vi "HFRR ADV v07.vi"() -> ()   [LabVIEW 2025] (continued)
    n1256 = property on="FF Calibration g" class="WFGraph (strict)"("Visible"=w1675) -> ()  [unwired: 2 in, 2 out]
    n1257 = property on="Lift" class="Bool (strict)"("Visible"=w1675) -> ()  [unwired: 2 in, 2 out]
    n1258 = property on="Threshold" class="DigNum (strict)"("Visible"=w1675) -> ()  [unwired: 2 in, 2 out]
    n1259 = property on="Time slide" class="Slide (strict)"("Visible"=w1675) -> ()  [unwired: 2 in, 2 out]
    n1260 = call "Elapsed Time2"("Time Target (s)"=w1686, "Auto Reset"=TRUE) -> ("Time has Elapsed"=w1676:bool)  [unwired: 10 in, 7 out]
    n1261 = case shown="True" w1676 {
      frame False {
        # "79.77669138"
        # "2.3554"
        n1262 = local read "FRIC. FORCE :"() -> (w1739:dbl)
        n1263 = local read "FF cal val"() -> (w1736:dbl[])
        n1264 = Multiply(x=w1739, y=79.77669138) -> (x*y=w1738:dbl)
        n1265 = Multiply(x=w1736, y=w1738) -> (x*y=→"FF Calibration g":dbl[])
        "Err Count" <- 0 ("y")
      }
      frame True {
        n1266 = stacked-sequence {
          frame #0 {
            n1267 = stacked-sequence {
              frame #0 {
                "Lift" <- TRUE ("Lift")
              }
            }
          }
          frame #1 {
            w1751 = 2500 ("y")
            n1268 = local read "RUN"() -> (w1743:bool)
            n1269 = local read "FF1"() -> (w1746:dbl[])
            n1270 = case shown="False" w1743 {
              frame False {
                n1271 = local write "Frequency"(0.0 ("Frequency")) -> ()
              }
              frame True {
              }
            }
            n1272 = Array Size(array=w1746) -> (size(s)=w1745:i32)
            n1273 = local read "Ch1"() -> (w1742:dbl[])
            "Waveform Chart 2" <- w1742
            n1274 = call-poly <vilib>:"Mean.vi"("X"=w1742) -> ("mean"=→"Raw Mean":dbl)  [unwired: 1 out]
            n1275 = Insert Into Array(array=w1746, index=w1745, new element=w1742) -> (w1748:dbl[])
            n1276 = Array Size(array=w1748) -> (size(s)=w1752:i32)
            n1277 = Subtract(x=w1752, y=w1751) -> (x-y=w1750:i32)
            n1278 = Greater?(x=w1752, y=w1751) -> (0:w1753:bool)
            n1279 = case shown="True" w1753 {
              tunnel: w1750 -> [_ w1757]
              tunnel: [w1755 w1759] -> w1744
              tunnel: w1748 -> [w1755 w1758]
              frame False {
              }
              frame True {
                n1280 = Delete From Array(array=w1758, length=w1757, index=0) -> (array with subset deleted=w1759:dbl[])  [unwired: 1 out]
                "Numeric" <- w1757
              }
            }
            "FF1" <- w1744
            "PID Ref" <- TRUE ("PID Ref")
          }
          frame #2 {
          }
          frame #3 {
            w1767 = 0.0 ("lower limit")
            # "CONVERT TO N"
            # "DATA PROCESSING"
            # "115 mV/N"
            n1281 = local read "RH Numeric:"() -> (w1761:dbl)
            n1282 = local read "HUMIDITY:"() -> (w1762:dbl)
            n1283 = local read "temp buf"() -> (w1825:dbl[])
            n1284 = local read "Air temp"() -> (w1823:dbl[])
            n1285 = local read "ecr buf"() -> (w1784:dbl[])
            n1286 = local read "Fric Val"() -> (w1829:dbl[])
            n1287 = case shown="True" "Boolean 5" {
              frame False {
              }
              frame True {
                n1288 = local write "Boolean 5"(FALSE) -> ()
                n1289 = local write "Captured Values"(dbl[][] [] ("Captured Values")) -> ()
                n1290 = local write "Best Fit"(dbl[] [] ("Best Fit")) -> ()
              }
            }
            n1291 = local read "TEMPERATURE :"() -> (w1806:dbl)
            n1292 = call-poly <vilib>:"Mean.vi"("X"=w1784) -> ("mean"=w1781:dbl)  [unwired: 1 out]
            n1293 = call-poly <vilib>:"Mean.vi"("X"=w1823) -> ("mean"=w1791:dbl)  [unwired: 1 out]
            "Raw air temp" <- w1791
            n1294 = call-poly <vilib>:"Mean.vi"("X"=w1825) -> ("mean"=w1793:dbl)  [unwired: 1 out]
            "Raw specimen temp" <- w1793
            n1295 = local read "TEMP INTERCEPT:"() -> (w1798:dbl)
            n1296 = Multiply(x=w1761, y=w1762) -> (x*y=→"Humidity ( %RH )" →"Hum" →"Hum 2":dbl)
            n1297 = Multiply(x=w1829, y=1.0) -> (x*y=w1830:dbl[])
            n1298 = local read "FRIC. FORCE :"() -> (w1822:dbl)
            n1299 = Multiply(x=w1793, y=w1806) -> (x*y=w1787:dbl)
            n1300 = local read "AIR TEMPERATURE :"() -> (w1807:dbl)
            n1301 = local read "RUN"() -> (w1819:bool)
            n1302 = Add(x=w1791, y="Offset Air Temp") -> (x+y=w1786:dbl)
            n1303 = local read "AIR TEMP INTERCEPT:"() -> (w1803:dbl)
            n1304 = case shown="0, Default" "Calibrating" {
              tunnel: w1793 -> [w1849 _]
              tunnel: [w1849 w1850] -> w1792
              tunnel: w1791 -> [_ w1850]
              frame 0, Default {
              }
              frame 1 {
              }
            }
            n1305 = Multiply(x=w1781, y="ECR_Gain") -> (x*y=w1780:dbl)
            n1306 = Add(x=w1787, y=w1798) -> (x+y=w1804:dbl)
            n1307 = Multiply(x=w1822, y=79.77669138) -> (x*y=w1820:dbl)
            n1308 = Select(t=0.01 ("FF fil1"), s=w1819, f=0.1 ("FF fil1")) -> (s? t:f=w1815:dbl)
            n1309 = local read "ecr"() -> (w1775:dbl)
            n1310 = Multiply(x=w1786, y=w1807) -> (x*y=w1788:dbl)
            n1311 = Multiply(x=w1830, y=w1820) -> (x*y=w1827:dbl[])
            n1312 = Multiply(x=w1780, y=0.2) -> (x*y=w1773:dbl)
            n1313 = Multiply(x=0.8, y=w1775) -> (x*y=w1774:dbl)
            n1314 = call <vilib>:"Mean PtByPt.vi"("x"=w1804, "sample length"=10) -> ("mean"=w1763:dbl)  [unwired: 2 in, 1 out]
            "TEMP 2" <- w1763
            "TEMP 3" <- w1763
            n1315 = local read "AIR TEMP"() -> (w1812:dbl)
            n1316 = Add(x=w1788, y=w1803) -> (x+y=w1805:dbl)
            n1317 = call-poly <vilib>:"Mean.vi"("X"=w1827) -> ("mean"=w1828:dbl)  [unwired: 1 out]
            n1318 = Add(x=w1773, y=w1774) -> (x+y=w1772:dbl)
            n1319 = Subtract(x=1.0 ("y"), y=w1815) -> (x-y=w1813:dbl)
            n1320 = local write "TEMP"(w1763) -> ()
            n1321 = Multiply(x=w1813, y=w1812) -> (x*y=w1811:dbl)
            n1322 = Multiply(x=w1805, y=w1815) -> (x*y=w1816:dbl)
            n1323 = Not A Number/Path/Refnum?(number/path/refnum=w1772) -> (NaN/Path/Refnum?=w1782:bool)
            n1324 = Subtract(x=w1827, y=w1828) -> (x-y=w1797:dbl[])
            n1325 = local read "FRICVALZ"() -> (w1837:dbl)
            n1326 = case shown="True" "Boolean 4" {
              tunnel: w1792 -> [_ w1856]
              tunnel: "Standard Temp. ( °c )" -> [_ w1855]
              frame False {
              }
              frame True {
                n1327 = Build Array(w1855, w1856) -> (w1854:dbl[])
                n1328 = local write "Boolean 4"(FALSE ("Boolean 4")) -> ()
                n1329 = local read "Captured Values"() -> (w1853:dbl[][])
                n1330 = Build Array (concatenate)(w1853, w1854) -> (w1851:dbl[][])
                n1331 = local write "Captured Values"(w1851) -> ()
              }
            }
            n1332 = Or(x="FRICVALZ 3", y="FRICVALZ 2") -> (x .or. y?=w1765:bool)
            n1333 = Add(x=w1816, y=w1811) -> (x+y=w1809:dbl)
            n1334 = Absolute Value(x=w1797) -> (abs(x)=w1832:dbl[])
            n1335 = call-poly <vilib>:"RMS.vi"("X"=w1797) -> ("rms value"=w1796:dbl)  [unwired: 1 out]
            n1336 = Select(t=0.0, s=w1782, f=w1772) -> (s? t:f=w1779:dbl)
            n1337 = call-poly <vilib>:"Mean.vi"("X"=w1832) -> ()  [unwired: 2 out]
            n1338 = local read "FF 2"() -> (w1839:dbl)
            n1339 = case shown="True" w1765 {
              tunnel: w1796 -> [_ w1861]
              frame False {
              }
              frame True {
                w1860 = FALSE ("FRICVALZ")
                n1340 = local write "FRICVALZ 3"(w1860) -> ()
                n1341 = local write "FRICVALZ 2"(w1860) -> ()
                "FRICVALZ" <- w1861
              }
            }
            n1342 = Subtract(x=w1796, y=w1837) -> (x-y=w1831:dbl)
            n1343 = Not A Number/Path/Refnum?(number/path/refnum=w1809) -> (NaN/Path/Refnum?=w1810:bool)
            n1344 = In Range and Coerce(upper limit=100.0, x=w1779, lower limit=w1767) -> ()  [unwired: 2 out]
            n1345 = Select(t=0.0, s=w1810, f=w1809) -> (s? t:f=w1769:dbl)
            "AIR TEMP" <- w1769
            n1346 = Multiply(x=w1831, y=0.1 ("FF fil1")) -> (x*y=w1843:dbl)
            n1347 = Multiply(x=0.9 ("FF fil2"), y=w1839) -> (x*y=w1842:dbl)
            n1348 = call "Elapsed Time11"("Time Target (s)"=1.0) -> ("Time has Elapsed"=w1771:bool)  [unwired: 11 in, 7 out]
            n1349 = Add(x=w1843, y=w1842) -> (x+y=w1766:dbl)
            "FF 2" <- w1766
            "FF 4" <- w1766
            n1350 = local read "NORMAL LOAD"() -> (w1826:dbl)
            n1351 = case shown="True" w1771 {
              tunnel: w1769 -> [_ w1845]
              frame False {
              }
              frame True {
                "AirT" <- w1845
              }
            }
            n1352 = local read "TEMP"() -> (w1836:dbl)
            n1353 = Not A Number/Path/Refnum?(number/path/refnum=w1766) -> (NaN/Path/Refnum?=w1834:bool)
            n1354 = Divide(x=w1766, y=w1826) -> (x/y=w1799:dbl)
            n1355 = Not A Number/Path/Refnum?(number/path/refnum=w1836) -> (NaN/Path/Refnum?=w1835:bool)
            n1356 = Compound Arithmetic op=OR(w1835, w1834) -> (w1833:bool)
            n1357 = Not A Number/Path/Refnum?(number/path/refnum=w1799) -> (NaN/Path/Refnum?=w1801:bool)
            n1358 = case shown="True" w1833 {
              frame False {
              }
              frame True {
                n1359 = local write "TEMP"(0.0 ("TEMP")) -> ()
                n1360 = local write "FF 2"(0.0 ("FF 2")) -> ()
                n1361 = local write "reinit"(TRUE ("reinit")) -> ()
              }
            }
            n1362 = Select(t=0.0, s=w1801, f=w1799) -> (s? t:f=→"COF 2":dbl)
            "ecr" <- w1767
          }
          frame #4 {
            n1363 = flat-sequence {
              frame #0 {
                n1364 = Wait (ms)(milliseconds to wait=u32 100) -> ()  [unwired: 1 out]
              }
              frame #1 {
                n1365 = local write "Lift"(FALSE ("Lift")) -> ()
              }
            }
            n1366 = case shown="True" "Boolean 6" {
              frame False {
              }
              frame True {
                n1367 = local write "Boolean 6"(FALSE ("Boolean 6")) -> ()
                n1368 = local read "Captured Values"() -> (w1872:dbl[][])
                n1369 = Index Array(array=w1872, index (col) #1=0 ("disabled index (col)"), index (col) #2=1 ("index (col)")) -> (element #1=w1870:dbl[], element #2=w1868:dbl[])  [unwired: 2 in]
                n1370 = call <vilib>:"Linear Fit.vi"("Y"=w1870, "X"=w1868) -> ("Best Linear Fit"=→"Best Fit":dbl[], "slope"=w1864:dbl, "intercept"=w1863:dbl)  [unwired: 9 in, 2 out]
                "Slope" <- w1864
                "Intercept" <- w1863
                n1371 = local read "Calibrating"() -> (w1865:u16)
                n1372 = case shown="1" w1865 {
                  tunnel: w1864 -> [w1874 w1876]
                  tunnel: w1863 -> [w1873 w1875]
                  frame 0, Default {
                    n1373 = local write "TEMPERATURE :"(w1874) -> ()
                    n1374 = local write "TEMP INTERCEPT:"(w1873) -> ()
                  }
                  frame 1 {
                    n1375 = local write "AIR TEMPERATURE :"(w1876) -> ()
                    n1376 = local write "AIR TEMP INTERCEPT:"(w1875) -> ()
                  }
                }
              }
            }
          }
        }
      }
    }
    n1377 = Wait (ms)(milliseconds to wait=u32 50) -> ()  [unwired: 1 out]
    n1378 = local read "Quit"() -> (w1667:bool)
    "Rate" <- 2500.0 ("No of Samples")
    "Humid Last buf" <- dbl[] [0.0, 0.0, 0.0, 0.0] ("Humid Last buf")
  }
  n1379 = while {
    tunnel: w53 -> [_]
    tunnel: [w1906] -> _
    tunnel: [w1881] -> w50
    i -> [w1906]
    stop <- w1881 stop-if-true
    # "C:\\LAB-IQ-NXT\\Scar View.exe"
    n1380 = local read "OK Button 16"() -> (w1895:bool)
    n1381 = local read "Re-Initialise"() -> (w1891:bool)
    n1382 = local read "Main Tab"() -> (w1887:T3)
    n1383 = local read "service 3"() -> (w1888:bool)
    n1384 = local read "OPEN 6"() -> (w1890:bool)
    n1385 = local read "EDIT 2"() -> (w1893:bool)
    n1386 = flat-sequence {
      frame #0 {
        n1387 = stacked-sequence {
          frame #0 {
            n1388 = local read "EDIT"() -> (w2560:bool)
            n1389 = case shown="True" w2560 {
              tunnel: [u8 2 ("Disabled") u8 0 ("Disabled")] -> _
              frame False {
                w2562 = FALSE
                n1390 = local write "Password"("") -> ()
                n1391 = property on="SrvM CP" class="Bool (strict)"("Visible"=w2562) -> ()  [unwired: 2 in, 2 out]
                n1392 = property on="message" class="Str"("Visible"=w2562) -> ()  [unwired: 2 in, 2 out]
                n1393 = local write "x = y?"(w2562) -> ()
                n1394 = property on="Password" class="Str"("Visible"=w2562) -> ()  [unwired: 2 in, 2 out]
                n1395 = property on="ENTER THE NEW PASSWORD" class="Str"("Visible"=w2562) -> ()  [unwired: 2 in, 2 out]
                n1396 = property on="ENTER CURRENT PASSWORD" class="Str"("Visible"=w2562) -> ()  [unwired: 2 in, 2 out]
                n1397 = local write "SrvM CP"(w2562) -> ()
              }
              frame True {
                w2565 = TRUE
                n1398 = property on="SrvM CP" class="Bool (strict)"("Visible"=w2565) -> ()  [unwired: 2 in, 2 out]
                n1399 = property on="Password" class="Str"("Visible"=w2565) -> ()  [unwired: 2 in, 2 out]
              }
            }
            "dipl pwd" <- "@143$\n" ("dipl pwd")
          }
          frame #1 {
            # "Gain password"
            n1400 = String To Byte Array(string="ENTER CURRENT PASSWORD") -> (unsigned byte array=w2570:u8[])
            n1401 = Search 1D Array(1D array=w2570, element=u8 10) -> (index of element=w2573:i32)  [unwired: 1 in]
            n1402 = Index Array(array=w2570, index=w2573) -> (element=w2569:u8)
            n1403 = Equal?(x=w2569, y=10) -> (x = y?=w2567:bool)
            n1404 = case shown="True" w2567 {
              frame False {
                n1405 = property on="ENTER THE NEW PASSWORD" class="Str"("Visible"=FALSE) -> ()  [unwired: 2 in, 2 out]
              }
              frame True {
                # "password"
                # "change password logic"
                n1406 = local read "ENTER CURRENT PASSWORD"() -> (w2586:string)
                n1407 = local read "dipl pwd"() -> (w2580:string)
                n1408 = String To Byte Array(string=w2586) -> (unsigned byte array=w2588:u8[])
                n1409 = String To Byte Array(string=w2580) -> (unsigned byte array=w2581:u8[])
                n1410 = Array Size(array=w2588) -> (size(s)=w2585:i32)
                n1411 = Array Size(array=w2581) -> (size(s)=w2583:i32)
                n1412 = for {
                  N: w2585 -> [_]
                  tunnel: w2588 -> [w2612]
                  tunnel: [w2610] -> w2589 mode=indexing
                  tunnel: w2585 -> [w2604]
                  i -> [w2605]
                  n1413 = Decrement(x=w2604) -> (x-1=w2602:i32)
                  n1414 = Equal?(x=w2605, y=w2602) -> (x = y?=w2603:bool)
                  n1415 = Index Array(array=w2612, index=w2605) -> (element=w2606:u8)
                  n1416 = Number To Decimal String(number=w2606) -> (decimal integer string=w2611:string)  [unwired: 1 in]
                  n1417 = Select(t="", s=w2603, f="\r") -> (s? t:f=w2608:string)
                  n1418 = Concatenate Strings(w2611, w2608) -> (w2610:string)
                }
                n1419 = for {
                  N: w2583 -> [_]
                  tunnel: w2581 -> [w2600]
                  tunnel: [w2598] -> w2582 mode=indexing
                  tunnel: w2583 -> [w2595]
                  i -> [w2596]
                  n1420 = Decrement(x=w2595) -> (x-1=w2594:i32)
                  n1421 = Equal?(x=w2596, y=w2594) -> (x = y?=w2593:bool)
                  n1422 = Index Array(array=w2600, index=w2596) -> (element=w2599:u8)
                  n1423 = Number To Decimal String(number=w2599) -> (decimal integer string=w2597:string)  [unwired: 1 in]
                  n1424 = Select(t="", s=w2593, f="\r") -> (s? t:f=w2590:string)
                  n1425 = Concatenate Strings(w2597, w2590) -> (w2598:string)
                }
                n1426 = local read "string"() -> (w2587:string)
                n1427 = Concatenate Strings(w2582) -> (w2576:string)
                n1428 = Concatenate Strings(w2587) -> (w2584:string)
                n1429 = Concatenate Strings(w2589) -> (w2577:string)
                n1430 = Equal?(x=w2577, y=w2584) -> (x = y?=w2579:bool)
                n1431 = Equal?(x=w2577, y=w2576) -> (x = y?=w2575:bool)
                n1432 = Or(x=w2579, y=w2575) -> (x .or. y?=w2578:bool)
                n1433 = case shown="True" w2578 {
                  frame False {
                  }
                  frame True {
                    n1434 = property on="ENTER THE NEW PASSWORD" class="Str"("Visible"=TRUE) -> ()  [unwired: 2 in, 2 out]
                  }
                }
              }
            }
          }
          frame #2 {
            n1435 = String To Byte Array(string="ENTER THE NEW PASSWORD") -> (unsigned byte array=w2615:u8[])
            n1436 = Search 1D Array(1D array=w2615, element=u8 10) -> (index of element=w2619:i32)  [unwired: 1 in]
            n1437 = Index Array(array=w2615, index=w2619) -> (element=w2617:u8)
            n1438 = Equal?(x=w2617, y=10) -> (x = y?=w2614:bool)
            n1439 = case shown="False" w2614 {
              frame False {
              }
              frame True {
                n1440 = local write "EDIT"(FALSE) -> ()
                n1441 = local write "SrvM CP"(FALSE) -> ()
                n1442 = local read "ENTER THE NEW PASSWORD"() -> (w2622:string)
                n1443 = String To Byte Array(string=w2622) -> (unsigned byte array=w2627:u8[])
                n1444 = Array Size(array=w2627) -> (size(s)=w2624:i32)
                n1445 = for {
                  N: w2624 -> [_]
                  tunnel: w2627 -> [w2640]
                  tunnel: [w2637] -> w2629 mode=indexing
                  tunnel: w2624 -> [w2632]
                  i -> [w2630]
                  n1446 = Decrement(x=w2632) -> (x-1=w2633:i32)
                  n1447 = Equal?(x=w2630, y=w2633) -> (x = y?=w2634:bool)
                  n1448 = Index Array(array=w2640, index=w2630) -> (element=w2639:u8)
                  n1449 = Number To Decimal String(number=w2639) -> (decimal integer string=w2638:string)  [unwired: 1 in]
                  n1450 = Select(t="", s=w2634, f="\r") -> (s? t:f=w2631:string)
                  n1451 = Concatenate Strings(w2638, w2631) -> (w2637:string)
                }
                n1452 = local read "file path"() -> (w2621:path)
                n1453 = Concatenate Strings(w2629) -> (w2623:string)
                n1454 = Delete(path (use dialog)=w2621) -> (deleted path=w2625:path)  [unwired: 4 in, 2 out]
                n1455 = call <vilib>:"Write Characters To File.vi"("append to file? (new file:F)"=FALSE, "character string"=w2623, "file path (dialog if empty)"=w2625) -> ()  [unwired: 2 in, 1 out]
              }
            }
          }
          frame #3 {
            n1456 = case shown="True" "SrvM CP" {
              frame False {
                w2643 = ""
                n1457 = local write "ENTER CURRENT PASSWORD"(w2643) -> ()
                n1458 = local write "ENTER THE NEW PASSWORD"(w2643) -> ()
                n1459 = property on="ENTER CURRENT PASSWORD" class="Str"("Visible"=FALSE) -> ()  [unwired: 2 in, 2 out]
              }
              frame True {
                n1460 = property on="ENTER THE NEW PASSWORD" class="Str"() -> ("Visible"=w2644:bool)  [unwired: 2 in, 2 out]
                n1461 = Not(x=w2644) -> (.not. x?=w2645:bool)
                n1462 = property on="ENTER CURRENT PASSWORD" class="Str"("Visible"=w2645) -> ()  [unwired: 2 in, 2 out]
              }
            }
          }
          frame #4 {
            n1463 = String To Byte Array(string="Password") -> (unsigned byte array=w2652:u8[])
            n1464 = Search 1D Array(1D array=w2652, element=u8 10) -> (index of element=w2650:i32)  [unwired: 1 in]
            n1465 = Index Array(array=w2652, index=w2650) -> (element=w2651:u8)
            n1466 = Equal?(x=w2651, y=10) -> (x = y?=w2647:bool)
            n1467 = case shown="True" w2647 {
              frame False {
              }
              frame True {
                # "password"
                # "password"
                n1468 = local read "Password"() -> (w2665:string)
                n1469 = String To Byte Array(string=w2665) -> (unsigned byte array=w2668:u8[])
                n1470 = String To Byte Array(string="@143$\n") -> (unsigned byte array=w2654:u8[])
                n1471 = Array Size(array=w2668) -> (size(s)=w2663:i32)
                n1472 = Array Size(array=w2654) -> (size(s)=w2659:i32)
                n1473 = for {
                  N: w2663 -> [_]
                  tunnel: w2668 -> [w2685]
                  tunnel: [w2683] -> w2669 mode=indexing
                  tunnel: w2663 -> [w2680]
                  i -> [w2681]
                  n1474 = Decrement(x=w2680) -> (x-1=w2679:i32)
                  n1475 = Index Array(array=w2685, index=w2681) -> (element=w2684:u8)
                  n1476 = Equal?(x=w2681, y=w2679) -> (x = y?=w2678:bool)
                  n1477 = Number To Decimal String(number=w2684) -> (decimal integer string=w2682:string)  [unwired: 1 in]
                  n1478 = Select(t="", s=w2678, f="\r") -> (s? t:f=w2675:string)
                  n1479 = Concatenate Strings(w2682, w2675) -> (w2683:string)
                }
                n1480 = for {
                  N: w2659 -> [_]
                  tunnel: w2654 -> [w2696]
                  tunnel: [w2694] -> w2657 mode=indexing
                  tunnel: w2659 -> [w2691]
                  i -> [w2692]
                  n1481 = Decrement(x=w2691) -> (x-1=w2690:i32)
                  n1482 = Index Array(array=w2696, index=w2692) -> (element=w2695:u8)
                  n1483 = Equal?(x=w2692, y=w2690) -> (x = y?=w2689:bool)
                  n1484 = Number To Decimal String(number=w2695) -> (decimal integer string=w2693:string)  [unwired: 1 in]
                  n1485 = Select(t="", s=w2689, f="\r") -> (s? t:f=w2686:string)
                  n1486 = Concatenate Strings(w2693, w2686) -> (w2694:string)
                }
                n1487 = local read "file path"() -> (w2653:path)
                n1488 = call <vilib>:"Read Characters From File.vi"("file path (dialog if empty)"=w2653) -> ("character string"=w2667:string)  [unwired: 5 in, 3 out]
                "string" <- w2667
                n1489 = flat-sequence {
                  tunnel: [w2670] -> w2664
                  frame #0 {
                    w2670 = ""
                    n1490 = local write "Password"(w2670) -> ()
                  }
                }
                n1491 = Concatenate Strings(w2657) -> (w2658:string)
                n1492 = Concatenate Strings(w2667) -> (w2666:string)
                n1493 = Concatenate Strings(w2669) -> (w2661:string)
                n1494 = Equal?(x=w2661, y=w2666) -> (x = y?=w2656:bool)
                n1495 = Equal?(x=w2661, y=w2658) -> (x = y?=w2662:bool)
                n1496 = Or(x=w2656, y=w2662) -> (x .or. y?=w2655:bool)
                "x = y?" <- w2655
                n1497 = case shown="False" w2655 {
                  selector: w2655 -> [w2672 _]
                  tunnel: w2664 -> [_ _]
                  frame False {
                    n1498 = And(x=w2672, y=TRUE ("Visible")) -> (x .and. y?=w2673:bool)
                    n1499 = property on="message" class="Str"("Visible"=w2673) -> ()  [unwired: 2 in, 2 out]
                  }
                  frame True {
                    n1500 = property on="message" class="Str"("Visible"=FALSE) -> ()  [unwired: 2 in, 2 out]
                  }
                }
              }
            }
          }
        }
        n1501 = local read "x = y?"() -> (w2512:bool)
        n1502 = local read "HUMIDITY: 2"() -> (w2514:dbl)
        n1503 = local read "HUMIDITY:"() -> (w2513:dbl)
        n1504 = property on="Port 2 Error" class="Clust (strict)"("Visible"="EDIT") -> ()  [unwired: 2 in, 2 out]
        n1505 = property on="Port 1 Error" class="Clust (strict)"("Visible"="EDIT") -> ()  [unwired: 2 in, 2 out]
        n1506 = case shown="True" "SrvM CP 2" {
          frame False {
          }
          frame True {
            n1507 = local write "SrvM CP 2"(FALSE ("SrvM CP 2")) -> ()
            n1508 = local read "HUMIDITY: 2"() -> (w2553:dbl)
            n1509 = local read "TEMP INTERCEPT: 2"() -> (w2552:dbl)
            n1510 = local read "DISPLACEMENT : 4"() -> (w2556:dbl)
            n1511 = local read "TEMPERATURE : 2"() -> (w2555:dbl)
            n1512 = local read "STROKE GAIN : 2"() -> (w2557:dbl)
            n1513 = local read "FRIC. FORCE : 2"() -> (w2558:dbl)
            n1514 = local read "AIR TEMP INTERCEPT: 2"() -> (w2551:dbl)
            n1515 = local read "AIR TEMPERATURE : 2"() -> (w2554:dbl)
            n1516 = local write "HUMIDITY:"(w2553) -> ()
            n1517 = local write "AIR TEMP INTERCEPT:"(w2552) -> ()
            n1518 = local write "TEMPERATURE :"(w2555) -> ()
            n1519 = local write "FRIC. FORCE :"(w2558) -> ()
            n1520 = local write "STROKE GAIN :"(w2557) -> ()
            n1521 = local write "DISPLACEMENT :"(w2556) -> ()
            n1522 = local write "AIR TEMPERATURE :"(w2554) -> ()
            n1523 = local write "TEMP INTERCEPT:"(w2551) -> ()
          }
        }
        n1524 = case shown="True" "SAVE" {
          frame False {
          }
          frame True {
            n1525 = stacked-sequence {
              seq-local: [w2713 _ _] -> [_ w2877 _]
              frame #0 {
                (unwired) i16 5 ("precision (6)")
                # "[CH1]    - FF\n[CH2]   - TEMPERATURE\n[CH3]    - Humidity\n[CH4]    - AIR TEMP\n[CH5]\\- Visa Uno\n[CH6] \\- Visa Due\n[CH7]  \\- file path\n[CH8]   - Displacement Gain\n[CHA]   - Stroke Gain\n[CHB]   - Stroke PID Gain\n[CHC]   -Language Selection\n[CHD]   -Power +\n[CHE]   -Power_\n[CHF]   -Heater\n[CHG]   -Humidity Wet\n[CHH]   -Humidity Dry\n[CHI]   -Integral Time"
                n1526 = local read "Stroke PID Gains"() -> (w2764:T9)
                n1527 = Unbundle By Name(w2764) -> ("Proportional Gain (Kc)"=w2763:dbl, "Integral Time (Ti, min)"=w2705:dbl)
                n1528 = Number To Fractional String(number=w2705, width (-)=i16 10 ("precision (6)"), precision (6)=i16 5) -> (F-format string=w2709:string)  [unwired: 1 in]
                n1529 = local read "Language Selection"() -> (w2761:enum16{"English", "Russian"})
                n1530 = local read "CH-HUMIDITY WET"() -> (w2719:u16)
                n1531 = local read "CH-HUMIDITY DRY"() -> (w2716:u16)
                n1532 = local read "STROKE GAIN :"() -> (w2697:dbl)
                n1533 = local read "CH-POWER +"() -> (w2728:u16)
                n1534 = local read "CH-POWER -"() -> (w2725:u16)
                n1535 = local read "CH-HEATER"() -> (w2722:u16)
                n1536 = local read "AIR TEMPERATURE :"() -> (w2700:dbl)
                n1537 = Concatenate Strings("[CHI]" ("string"), w2709, "-Integral Time " ("string"), "\r") -> (w2706:string)
                n1538 = local read "DISPLACEMENT :"() -> (w2698:dbl)
                n1539 = local read "TEMPERATURE :"() -> (w2701:dbl)
                n1540 = local read "FRIC. FORCE :"() -> (w2702:dbl)
                n1541 = local read "HUMIDITY:"() -> (w2699:dbl)
                n1542 = Path To String(path="File Path") -> (string=w2786:string)
                n1543 = Number To Fractional String(number=w2697, width (-)=i16 10 ("precision (6)"), precision (6)=i16 5) -> (F-format string=w2777:string)  [unwired: 1 in]
                n1544 = Number To Fractional String(number=w2763, width (-)=i16 10 ("precision (6)"), precision (6)=i16 5) -> (F-format string=w2765:string)  [unwired: 1 in]
                n1545 = Number To Fractional String(number=w2761, width (-)=i16 10 ("precision (6)"), precision (6)=i16 5) -> (F-format string=w2757:string)  [unwired: 1 in]
                n1546 = Number To Fractional String(number=w2728, width (-)=i16 10 ("precision (6)"), precision (6)=i16 5) -> (F-format string=w2751:string)  [unwired: 1 in]
                n1547 = Number To Fractional String(number=w2725, width (-)=i16 10 ("precision (6)"), precision (6)=i16 5) -> (F-format string=w2748:string)  [unwired: 1 in]
                n1548 = Number To Fractional String(number=w2722, width (-)=i16 10 ("precision (6)"), precision (6)=i16 5) -> (F-format string=w2743:string)  [unwired: 1 in]
                n1549 = Number To Fractional String(number=w2719, width (-)=i16 10 ("precision (6)"), precision (6)=i16 5) -> (F-format string=w2740:string)  [unwired: 1 in]
                n1550 = Number To Fractional String(number=w2716, width (-)=i16 10 ("precision (6)"), precision (6)=i16 5) -> (F-format string=w2735:string)  [unwired: 1 in]
                n1551 = local read "Com Port 1"() -> (w2704:refnum<visa-resource-name>)
                n1552 = local read "Com Port 2"() -> (w2703:refnum<visa-resource-name>)
                n1553 = Concatenate Strings(w2786, "\\" ("string")) -> (w2785:string)
                n1554 = Number To Fractional String(number=w2702, width (-)=i16 10 ("precision (6)"), precision (6)=i16 5) -> (F-format string=w2818:string)  [unwired: 1 in]
                n1555 = Number To Fractional String(number=w2701, width (-)=i16 10 ("precision (6)"), precision (6)=i16 5) -> (F-format string=w2817:string)  [unwired: 1 in]
                n1556 = Number To Fractional String(number=w2699, width (-)=i16 10 ("precision (6)"), precision (6)=i16 5) -> (F-format string=w2811:string)  [unwired: 1 in]
                n1557 = Number To Fractional String(number=w2700, width (-)=i16 10 ("precision (6)"), precision (6)=i16 5) -> (F-format string=w2805:string)  [unwired: 1 in]
                n1558 = Number To Fractional String(number=w2698, width (-)=i16 10 ("precision (6)"), precision (6)=i16 5) -> (F-format string=w2778:string)  [unwired: 1 in]
                n1559 = Concatenate Strings("[CHA]" ("string"), w2777, "- Stroke Gain" ("string"), "\r") -> (w2771:string)
                n1560 = Concatenate Strings("[CHB]" ("string"), w2765, "- Stroke PID Gain" ("string"), "\r") -> (w2762:string)
                n1561 = Concatenate Strings("[CHC]" ("string"), w2757, "-Language Selection" ("string"), "\r") -> (w2754:string)
                n1562 = Concatenate Strings("[CHD]" ("string"), w2751, "-Power +" ("string"), "\r") -> (w2733:string)
                n1563 = Concatenate Strings("[CHG]" ("string"), w2740, "-Humidity Wet" ("string"), "\r") -> (w2730:string)
                n1564 = Concatenate Strings("[CHH]" ("string"), w2735, "-Humidity Dry" ("string"), "\r") -> (w2729:string)
                n1565 = Concatenate Strings("[CH1]" ("string"), w2818, " - FF" ("string"), "\r") -> (w2816:string)
                n1566 = Concatenate Strings("[CH2]" ("string"), w2817, " - TEMPERATURE" ("string"), "\r") -> (w2815:string)
                n1567 = Concatenate Strings("[CH3]" ("string"), w2811, " - Humidity" ("string"), "\r") -> (w2808:string)
                n1568 = Concatenate Strings("[CH4]" ("string"), w2805, " - AIR TEMP" ("string"), "\r") -> (w2801:string)
                n1569 = Concatenate Strings("[CH5]" ("string"), w2704, "- Visa Uno" ("string"), "\r") -> (w2794:string)
                n1570 = Concatenate Strings("[CH6]" ("string"), w2703, "- Visa Due" ("string"), "\r") -> (w2789:string)
                n1571 = Concatenate Strings("[CH7]" ("string"), w2785, "- file path" ("string"), "\r") -> (w2788:string)
                n1572 = Concatenate Strings("[CH8]" ("string"), w2778, "- Displacement Gain" ("string"), "\r") -> (w2781:string)
                n1573 = Concatenate Strings("[CHE]" ("string"), w2748, "-Power_" ("string"), "\r") -> (w2732:string)
                n1574 = Concatenate Strings("[CHF]" ("string"), w2743, "-Heater" ("string"), "\r") -> (w2731:string)
                n1575 = Concatenate Strings(w2816, w2815, w2808, w2801, w2794, w2789, w2788, w2781, w2771, w2762, w2754, w2733, w2732, w2731, w2730, w2729, w2706) -> (w2713:string)
                "gain" <- w2713
              }
              frame #1 {
                n1576 = local read "Camera Port :"() -> (w2830:string)
                n1577 = local read "TEMP INTERCEPT:"() -> (w2839:dbl)
                n1578 = local read "Humidity :"() -> (w2838:refnum<visa-resource-name>)
                n1579 = local read "AIR TEMP INTERCEPT:"() -> (w2840:dbl)
                n1580 = local read "LvdtOff"() -> (w2842:dbl)
                n1581 = Number To Fractional String(number=w2839, width (-)=i16 10 ("precision (6)"), precision (6)=i16 5) -> (F-format string=w2865:string)  [unwired: 1 in]
                n1582 = local read "Com Port 3"() -> (w2849:refnum<visa-resource-name>)
                n1583 = Concatenate Strings("[CH8]" ("string"), w2830, "- Visa Camera" ("string"), "\r") -> (w2829:string)
                n1584 = Concatenate Strings("[CH7]" ("string"), w2838, "- Visa Humidity" ("string"), "\r") -> (w2834:string)
                n1585 = Number To Fractional String(number=w2840, width (-)=i16 10 ("precision (6)"), precision (6)=i16 5) -> (F-format string=w2872:string)  [unwired: 1 in]
                n1586 = Number To Fractional String(number=w2842, width (-)=i16 10 ("precision (6)"), precision (6)=i16 5) -> (F-format string=w2846:string)  [unwired: 1 in]
                n1587 = Concatenate Strings("[CHK]" ("string"), w2865, "-TEMP INTERCEPT" ("string"), "\r") -> (w2861:string)
                n1588 = Concatenate Strings("[SNO]" ("string"), "S.NO", "-" ("string"), "\r") -> (w2857:string)
                n1589 = Concatenate Strings("[CHI]" ("string"), w2846, "-LVDT Position Offset" ("string"), "\r") -> (w2841:string)
                n1590 = Concatenate Strings("[CHJ]" ("string"), w2872, "-AIR TEMP INTERCEPT" ("string"), "\r") -> (w2862:string)
                n1591 = Concatenate Strings("[CHL]" ("string"), w2849, "- Visa humid" ("string"), "\r") -> (w2852:string)
                n1592 = String To Path(string="C:\\LAB-IQ\\calibrate WO 2465.dcf") -> (path=w2850:path)
                n1593 = Concatenate Strings(w2877, w2862, w2861, w2857, w2852, w2841, w2834, w2829) -> (w2876:string)
                n1594 = call <vilib>:"Write Characters To File.vi"("append to file? (new file:F)"=FALSE, "character string"=w2876, "file path (dialog if empty)"=w2850) -> ()  [unwired: 2 in, 1 out]
              }
              frame #2 {
                n1595 = local write "Lan flag"(0.0 ("Lan flag")) -> ()
                n1596 = local write "conststatus"(0.0 ("rpm value : 2")) -> ()
                n1597 = local write "SAVE"(FALSE ("OK Button 14")) -> ()
                n1598 = local write "Re-Initialise"(TRUE ("Re-Initialise")) -> ()
              }
            }
          }
        }
        n1599 = And(x="EDIT", y=w2512) -> (x .and. y?=w2510:bool)
        n1600 = local read "DISPLACEMENT : 4"() -> (w2523:dbl)
        n1601 = local read "TEMPERATURE : 2"() -> (w2521:dbl)
        n1602 = local read "STROKE GAIN : 2"() -> (w2527:dbl)
        n1603 = local read "DISPLACEMENT :"() -> (w2522:dbl)
        n1604 = local read "FRIC. FORCE : 2"() -> (w2530:dbl)
        n1605 = local read "TEMPERATURE :"() -> (w2519:dbl)
        n1606 = local read "STROKE GAIN :"() -> (w2526:dbl)
        n1607 = local read "FRIC. FORCE :"() -> (w2529:dbl)
        n1608 = case shown="False" w2510 {
          tunnel: [u8 2 ("Disabled") u8 0 ("Disabled")] -> w2509
          tunnel: [w2882 TRUE ("Visible")] -> w2508
          frame False {
            w2882 = FALSE ("Visible")
            n1609 = local write "EDIT 2"(w2882) -> ()
          }
          frame True {
          }
        }
        n1610 = Subtract(x=w2514, y=w2513) -> (x-y=w2515:dbl)
        n1611 = local read "AIR TEMPERATURE : 2"() -> (w2518:dbl)
        n1612 = local read "AIR TEMPERATURE :"() -> (w2517:dbl)
        n1613 = Divide(x=w2515, y=w2513) -> (x/y=w2537:dbl)
        n1614 = Subtract(x=w2530, y=w2529) -> (x-y=w2528:dbl)
        n1615 = Subtract(x=w2521, y=w2519) -> (x-y=w2520:dbl)
        n1616 = Subtract(x=w2527, y=w2526) -> (x-y=w2525:dbl)
        n1617 = Subtract(x=w2523, y=w2522) -> (x-y=w2524:dbl)
        n1618 = Subtract(x=w2518, y=w2517) -> (x-y=w2516:dbl)
        n1619 = Divide(x=w2528, y=w2529) -> (x/y=w2548:dbl)
        n1620 = Divide(x=w2520, y=w2519) -> (x/y=w2541:dbl)
        n1621 = Divide(x=w2525, y=w2526) -> (x/y=w2545:dbl)
        n1622 = Divide(x=w2524, y=w2522) -> (x/y=w2544:dbl)
        n1623 = Multiply(x=w2537, y=100.0) -> (x*y=→"HUMIDITY  Calibration Error":dbl)
        n1624 = Divide(x=w2516, y=w2517) -> (x/y=w2540:dbl)
        n1625 = Multiply(x=w2548, y=100.0) -> (x*y=→"FRIC. FORCE Calibration Error":dbl)
        n1626 = Multiply(x=w2541, y=100.0) -> (x*y=→"TEMPERATURE  Calibration Error":dbl)
        n1627 = Multiply(x=w2545, y=100.0) -> (x*y=→"STROKE Calibration Error":dbl)
        n1628 = Multiply(x=w2544, y=100.0) -> (x*y=→"DISPLACEMENT  Calibration Error":dbl)
        n1629 = property on="EDIT 2" class="Bool (strict)"("Visible"=w2508) -> ()  [unwired: 2 in, 2 out]
        n1630 = property on="SAVE" class="Bool (strict)"("Visible"=w2508) -> ()  [unwired: 2 in, 2 out]
        n1631 = property on="SrvM CP" class="Bool (strict)"("Disabled"=w2509) -> ()  [unwired: 2 in, 2 out]
        n1632 = property on="visa due" class="CmbBox"("Disabled"=w2509) -> ()  [unwired: 2 in, 2 out]
        n1633 = property on="LvdtOff" class="DigNum (strict)"("Disabled"=w2509) -> ()  [unwired: 2 in, 2 out]
        n1634 = property on="File Path" class="Path"("Disabled"=w2509) -> ()  [unwired: 2 in, 2 out]
        n1635 = Multiply(x=w2540, y=100.0) -> (x*y=→"AIR TEMPERATURE  Calibration Error":dbl)
        n1636 = property on="Tab Control" class="TabCtl (strict)"("Visible"=w2508) -> ()  [unwired: 2 in, 2 out]
        n1637 = property on="Language Selection" class="Enum (strict)"("Visible"=w2508) -> ()  [unwired: 2 in, 2 out]
        n1638 = property on="Tab Control 7" class="TabCtl (strict)"("Disabled"=w2509) -> ()  [unwired: 2 in, 2 out]
        n1639 = property on="AIR TEMP INTERCEPT:" class="DigNum (strict)"("Disabled"=w2509) -> ()  [unwired: 2 in, 2 out]
        n1640 = property on="CH-POWER -" class="DigNum (strict)"("Disabled"=w2509) -> ()  [unwired: 2 in, 2 out]
        n1641 = property on="CH-POWER +" class="DigNum (strict)"("Disabled"=w2509) -> ()  [unwired: 2 in, 2 out]
        n1642 = property on="AIR TEMPERATURE :" class="DigNum (strict)"("Disabled"=w2509) -> ()  [unwired: 2 in, 2 out]
        n1643 = property on="STROKE GAIN :" class="DigNum (strict)"("Disabled"=w2509) -> ()  [unwired: 2 in, 2 out]
        n1644 = property on="SPEED OUT:" class="DigNum (strict)"("Disabled"=w2509) -> ()  [unwired: 2 in, 2 out]
        n1645 = property on="CH-HUMIDITY DRY" class="DigNum (strict)"("Disabled"=w2509) -> ()  [unwired: 2 in, 2 out]
        n1646 = property on="HUMIDITY:" class="DigNum (strict)"("Disabled"=w2509) -> ()  [unwired: 2 in, 2 out]
        n1647 = property on="CH-HUMIDITY WET" class="DigNum (strict)"("Disabled"=w2509) -> ()  [unwired: 2 in, 2 out]
        n1648 = property on="Stroke PID Gains" class="Clust (strict)"("Disabled"=w2509) -> ()  [unwired: 2 in, 2 out]
        n1649 = property on="TEMPERATURE :" class="DigNum (strict)"("Disabled"=w2509) -> ()  [unwired: 2 in, 2 out]
        n1650 = property on="DISPLACEMENT :" class="DigNum (strict)"("Disabled"=w2509) -> ()  [unwired: 2 in, 2 out]
        n1651 = property on="CH-HEATER" class="DigNum (strict)"("Disabled"=w2509) -> ()  [unwired: 2 in, 2 out]
        n1652 = property on="TEMP INTERCEPT:" class="DigNum (strict)"("Disabled"=w2509) -> ()  [unwired: 2 in, 2 out]
        n1653 = property on="FRIC. FORCE :" class="DigNum (strict)"("Disabled"=w2509) -> ()  [unwired: 2 in, 2 out]
      }
    }
    n1654 = local read "RUN"() -> (w1905:bool)
    n1655 = local read "RUN"() -> (w1903:bool)
    n1656 = disable-structure shown="Disabled" {
      disable-tunnel: [w1920 _] -> w1885
      disable-tunnel: [w1919 _] -> w1883
      frame Disabled {
        n1657 = local read "Temperature before test"() -> (w1913:dbl)
        n1658 = local read "Temperature after test"() -> (w1926:dbl)
        n1659 = case shown="True" "Save Results" {
          frame False {
          }
          frame True {
            w1942 = "\r"
            n1660 = local write "Save Results"(FALSE ("OK Button 5")) -> ()
            n1661 = local read "Temperature before test"() -> (w1980:dbl)
            n1662 = local read "Temperature after test"() -> (w1982:dbl)
            n1663 = local read "Humidity before test"() -> (w1979:dbl)
            n1664 = local read "Humidity after test"() -> (w1981:dbl)
            n1665 = local read "WS1.4"() -> (w1986:dbl)
            n1666 = local read "AVP"() -> (w1984:dbl)
            n1667 = Number To Fractional String(number=w1986, width (-)=i16 6, precision (6)=i16 1) -> (F-format string=w1946:string)  [unwired: 1 in]
            n1668 = local read "MWSD"() -> (w1983:dbl)
            n1669 = local read "String"() -> (w1975:string)
            n1670 = local read "FILE"() -> (w1978:string)
            n1671 = local read "HCF"() -> (w1985:dbl)
            n1672 = Number To Fractional String(number=w1979, width (-)=i16 6, precision (6)=i16 1) -> (F-format string=w1971:string)  [unwired: 1 in]
            n1673 = Number To Fractional String(number=w1980, width (-)=i16 6, precision (6)=i16 1) -> (F-format string=w1968:string)  [unwired: 1 in]
            n1674 = Number To Fractional String(number=w1981, width (-)=i16 6, precision (6)=i16 1) -> (F-format string=w1964:string)  [unwired: 1 in]
            n1675 = Number To Fractional String(number=w1982, width (-)=i16 6, precision (6)=i16 1) -> (F-format string=w1960:string)  [unwired: 1 in]
            n1676 = Number To Fractional String(number=w1984, width (-)=i16 6, precision (6)=i16 3) -> (F-format string=w1953:string)  [unwired: 1 in]
            n1677 = Concatenate Strings(w1975, w1978) -> (w1997:string)
            n1678 = Number To Fractional String(number=w1983, width (-)=i16 6, precision (6)=i16 1) -> (F-format string=w1957:string)  [unwired: 1 in]
            n1679 = Number To Fractional String(number=w1985, width (-)=i16 6, precision (6)=i16 2) -> (F-format string=w1951:string)  [unwired: 1 in]
            n1680 = Concatenate Strings("(" ("string"), w1946, ")Microns" ("string")) -> (w1945:string)
            n1681 = local read "REMARKS"() -> (w1977:string)
            "REMARKS 2" <- w1977
            n1682 = Concatenate Strings("(" ("string"), w1971, " ) % RH," ("string")) -> (w1972:string)
            n1683 = Concatenate Strings(w1951, ")" ("string")) -> (w1949:string)
            n1684 = Concatenate Strings("(" ("string"), w1968, ")  Deg C ," ("string")) -> (w1967:string)
            n1685 = Concatenate Strings("(" ("string"), w1964, " ) % RH," ("string")) -> (w1963:string)
            n1686 = Concatenate Strings("(" ("string"), w1960, ")  Deg C ," ("string")) -> (w1959:string)
            n1687 = Concatenate Strings("(" ("string"), w1957, ")  Microns," ("string")) -> (w1956:string)
            n1688 = Concatenate Strings("(" ("string"), w1953, ")  kPa," ("string")) -> (w1943:string)
            n1689 = Concatenate Strings(w1997, ".dwm" ("Substring")) -> (w1995:string)
            n1690 = String To Path(string=w1995) -> (path=w1994:path)
            n1691 = Concatenate Strings(w1977, w1942, " Humidity before test= " ("Substring"), w1972, w1942, " Temperature before test = " ("Substring"), w1967, w1942, " Humidity after test= " ("Substring"), w1963, w1942, "Temperature after test = " ("Substring"), w1959, w1942, "MSD = " ("Substring"), w1956, w1942, "  AVP = " ("Substring"), w1943, w1942, "  HCF                     =( " ("Substring"), w1949, w1942, " WS1.4                  = " ("Substring"), w1945, w1942) -> (w1941:string)
            "data" <- w1941
            n1692 = call <vilib>:"Write Characters To File.vi"("append to file? (new file:F)"=FALSE, "character string"=w1941, "file path (dialog if empty)"=w1994) -> ()  [unwired: 2 in, 1 out]
            n1693 = Match Pattern(string=w1941, regular expression="!") -> (after substring=→"export":string)  [unwired: 1 in, 3 out]
          }
        }
        n1694 = Add(x=231.864, y=w1913) -> (x+y=w1910:dbl)
        n1695 = Add(x=231.864, y=w1926) -> (x+y=w1923:dbl)
        n1696 = Divide(x=1705.984, y=w1910) -> (x/y=w1911:dbl)
        n1697 = Divide(x=1705.984, y=w1923) -> (x/y=w1924:dbl)
        n1698 = local read "Humidity before test"() -> (w1915:dbl)
        n1699 = local read "Humidity after test"() -> (w1928:dbl)
        n1700 = Subtract(x=8.017352 ("y"), y=w1911) -> (x-y=w1937:dbl)
        n1701 = Subtract(x=8.017352 ("y"), y=w1924) -> (x-y=w1931:dbl)
        n1702 = expression code="10**y"(w1937) -> (w1917:dbl)
        n1703 = expression code="10**y"(w1931) -> (w1930:dbl)
        n1704 = Multiply(x=w1915, y=w1917) -> (x*y=w1916:dbl)
        n1705 = Multiply(x=w1928, y=w1930) -> (x*y=w1929:dbl)
        n1706 = Divide(x=w1916, y=750.0) -> (x/y=w1932:dbl)
        n1707 = Divide(x=w1929, y=750.0) -> (x/y=w1933:dbl)
        n1708 = Add(x=w1932, y=w1933) -> (x+y=w1934:dbl)
        n1709 = Divide(x=w1934, y=2.0) -> (x/y=w1936:dbl)
        n1710 = local write "AVP"(w1936) -> ()
        n1711 = Subtract(x=1.4, y=w1936) -> (x-y=w1919:dbl)
        n1712 = local read "HCF"() -> (w1920:dbl)
      }
      frame Enabled {
      }
    }
    n1713 = case shown="True" "EDIT 3" {
      frame False {
      }
      frame True {
        n1714 = local write "EDIT 3"(FALSE ("EDIT 3")) -> ()
        n1715 = local write "Main Tab"(T3."About" ("Main Tab")) -> ()
      }
    }
    n1716 = case shown="True" w1891 {
      frame False {
      }
      frame True {
        n1717 = local write "Re-Initialise"(FALSE ("Re-Initialise")) -> ()
      }
    }
    n1718 = case shown="False" w1905 {
      frame False {
        n1719 = local read "stopT"() -> (w2891:bool)
        n1720 = case shown="True" w2891 {
          frame False {
          }
          frame True {
            w2892 = FALSE
            n1721 = local write "stopT"(w2892) -> ()
            n1722 = local write "st enable"(w2892) -> ()
          }
        }
      }
      frame True {
        "stopT" <- TRUE
      }
    }
    n1723 = case shown="True" w1903 {
      frame False {
      }
      frame True {
        n1724 = local read "Main Tab"() -> (w2889:T3)
        n1725 = case shown="\"Compare Files\"" w2889 {
          frame "Acquire", Default {
          }
          frame "Compare Files" {
            n1726 = local write "Main Tab"(T3."Acquire" ("Main Tab")) -> ()
          }
          frame "About" {
          }
        }
      }
    }
    n1727 = case shown="True" w1893 {
      frame False {
        n1728 = property on="Password 2" class="Str"("Visible"=FALSE) -> ()  [unwired: 2 in, 2 out]
        n1729 = local write "Password 2"("" ("Password")) -> ()
      }
      frame True {
        n1730 = property on="Password 2" class="Str"("Visible"=TRUE) -> ()  [unwired: 2 in, 2 out]
        n1731 = Equal?(x="Password 2", y="HFRR1234") -> (x = y?=w2026:bool)
        n1732 = case shown="True" w2026 {
          tunnel: "Password 2" -> [w2029 _]
          frame False {
            n1733 = String Length(string=w2029) -> (length=w2030:i32)
            n1734 = Greater Than 0?(x=w2030) -> (x > 0?=w2028:bool)
            n1735 = case shown="False" w2028 {
              frame False {
                n1736 = property on="Password 2" class="Str"("Caption.Text"="Password (Advance Setting)") -> ()  [unwired: 2 in, 2 out]
              }
              frame True {
                n1737 = property on="Password 2" class="Str"("Caption.Text"="Incorrect Password!") -> ()  [unwired: 2 in, 2 out]
              }
            }
          }
          frame True {
            n1738 = local write "EDIT 2"(FALSE ("EDIT 2")) -> ()
            n1739 = local write "Password 2"("" ("Password")) -> ()
            n1740 = local write "Main Tab"(T3."Advance" ("Main Tab")) -> ()
          }
        }
      }
    }
    n1741 = case shown="True" "Prog Uno" {
      frame False {
      }
      frame True {
        n1742 = stacked-sequence {
          frame #0 {
            n1743 = Delete(path (use dialog)=path "C:/LAB-IQ-NXT/UNOCOMPILE.bat" ("working directory")) -> ()  [unwired: 4 in, 3 out]
          }
          frame #1 {
            n1744 = local read "Com Port 1"() -> (w2490:refnum<visa-resource-name>)
            n1745 = Concatenate Strings("cmd.exe /c \"mode " ("command line"), w2490, ":1200,n,8,1\"\n" ("command line")) -> (w2495:string)
            n1746 = Concatenate Strings(w2495, "CD\\\nCD WinDucom\navrdude -C avrdude.conf -v -patmega328p -carduino -P" ("command line"), w2490, " -b115200 -D -Uflash:w:UNO_V20.hex:i\n" ("command line"), "\r") -> (w2497:string)
            "STR" <- w2497
            n1747 = call <vilib>:"Write Characters To File.vi"("append to file? (new file:F)"=FALSE, "character string"=w2497, "file path (dialog if empty)"=path "C:/LAB-IQ/UNOCOMPILE.bat" ("working directory")) -> ()  [unwired: 2 in, 1 out]
          }
          frame #2 {
            n1748 = disable-structure shown="Disabled" {
              frame Disabled {
                w2501 = "cmd.exe  /c \"C:\\LAB-IQ-NXT\\UNOCOMPILE.bat\"" ("string")
                n1749 = local write "Prog Uno"(FALSE ("run minimized? (F)")) -> ()
                n1750 = call <vilib>:"System Exec.vi"("expected output size  (4096)"=u32 65535, "run minimized? (F)"=FALSE, "wait until completion? (T)"=TRUE ("run minimized? (F)"), "working directory"=path "C:/LAB-IQ-NXT", "standard input"=w2501, "command line"=w2501) -> ("error out"=w2500:errorcluster, "standard output"=→"String 42":string)  [unwired: 2 in, 2 out]
                "error out 3" <- w2500
                n1751 = flat-sequence {
                  tunnel: w2500 -> [_]
                  frame #0 {
                  }
                }
              }
              frame Enabled {
              }
            }
          }
        }
      }
    }
    n1752 = case shown="\"ASTM D6079\", Default" "TEST STANDARD" {
      tunnel: [2.0 ("Set Temp") 0.0 ("Set Temp") 2.0 ("Set Temp") 0.0 ("Set Temp")] -> w1894
      frame "ASTM D6079", Default {
        w2447 = 50.0 ("Hz")
        w2448 = 53.0 ("Set Rh")
        w2450 = 1.0 ("Set Strk")
        w2449 = 60.0 ("Set Temp")
        # "astm hide"
        n1753 = local write "NORMAL LOAD"(2.0 ("NORMAL LOAD")) -> ()
        n1754 = local write "Set Strk"(w2450) -> ()
        n1755 = local write "Set Hz"(w2447) -> ()
        n1756 = local write "Set Temp"(w2449) -> ()
        n1757 = local write "Set Rh"(w2448) -> ()
        n1758 = local write "test time"(75.0 ("test time")) -> ()
        n1759 = local write "Set Stroke:"(w2450) -> ()
        n1760 = local write "Set Humidity:"(w2448) -> ()
        n1761 = local write "Set Frequency:"(w2447) -> ()
        n1762 = local write "Set Temperature:"(w2449) -> ()
        "Test Standard" <- "ASTM D6079" ("Test Standard 2")
      }
      frame "ISO 12156" {
        n1763 = local write "Set Strk"(1.0 ("Set Strk")) -> ()
        n1764 = local write "NORMAL LOAD"(2.0 ("NORMAL LOAD")) -> ()
        n1765 = local write "Set Temp"(60.0 ("Set Temp")) -> ()
        n1766 = local write "test time"(75.0 ("test time")) -> ()
        n1767 = local write "Set Hz"(50.0 ("Hz")) -> ()
        n1768 = local write "Set Rh"(53.0 ("Set Rh")) -> ()
      }
      frame "CEC F-096-A-06" {
        n1769 = local write "Set Strk"(1.0 ("Set Strk")) -> ()
        n1770 = local write "NORMAL LOAD"(2.0 ("NORMAL LOAD")) -> ()
        n1771 = local write "Set Temp"(60.0 ("Set Temp")) -> ()
        n1772 = local write "test time"(75.0 ("test time")) -> ()
        n1773 = local write "Set Hz"(50.0 ("Hz")) -> ()
        n1774 = local write "Set Rh"(53.0 ("Set Rh")) -> ()
      }
      frame "Custom" {
      }
    }
    n1775 = case shown="True" "Prog Due" {
      frame False {
      }
      frame True {
        n1776 = stacked-sequence {
          frame #0 {
            n1777 = Delete(path (use dialog)=path "C:/LAB-IQ/DUECOMPILE.bat" ("working directory")) -> ()  [unwired: 4 in, 3 out]
          }
          frame #1 {
            n1778 = disable-structure shown="Disabled" {
              frame Disabled {
                n1779 = local read "visa due"() -> (w2472:string)
                n1780 = Concatenate Strings("cmd.exe /c \"mode " ("command line"), w2472, ":1200,n,8,1\"\n" ("command line")) -> (w2477:string)
                n1781 = Concatenate Strings(w2477, "CD\\\nCD WinDucom\nTIMEOUT 1\n bossac.exe -i -d --port=" ("command line"), w2472, " -U false -e -w -v -b DUE.bin -R\n" ("command line"), "\r") -> (w2479:string)
                "concatenated string 2" <- w2479
                n1782 = call <vilib>:"Write Characters To File.vi"("append to file? (new file:F)"=FALSE, "character string"=w2479, "file path (dialog if empty)"=path "C:/LAB-IQ-NXT/DUECOMPILE.bat" ("working directory")) -> ()  [unwired: 2 in, 1 out]
              }
              frame Enabled {
              }
            }
          }
          frame #2 {
            # "C:\\LAB-IQ-NXT\\DUECOMPILE.bat"
            n1783 = disable-structure shown="Disabled" {
              frame Disabled {
                w2484 = "cmd.exe  /c \"C:\\LAB-IQ-NXT\\DUECOMPILE.bat\"" ("string")
                n1784 = call <vilib>:"System Exec.vi"("expected output size  (4096)"=u32 65535, "run minimized? (F)"=FALSE, "wait until completion? (T)"=TRUE ("run minimized? (F)"), "working directory"=path "C:/LAB-IQ-NXT", "standard input"=w2484, "command line"=w2484) -> ("error out"=w2483:errorcluster, "standard output"=→"String 44":string)  [unwired: 2 in, 2 out]
                "error out 4" <- w2483
                n1785 = flat-sequence {
                  tunnel: w2483 -> [_]
                  frame #0 {
                  }
                }
              }
              frame Enabled {
              }
            }
            n1786 = local write "Prog Due"(FALSE ("Prog Due")) -> ()
          }
        }
      }
    }
    n1787 = Or(x=w1890, y=w1888) -> (x .or. y?=w1889:bool)
    n1788 = case shown="\"About\"" w1887 {
      tunnel: [T19."Acquire" ("Main Tab") T19."Compare Files" ("Main Tab") T19."About" ("Main Tab")] -> w1901
      frame "Acquire", Default {
      }
      frame "Compare Files" {
      }
      frame "About" {
      }
    }
    n1789 = Or(x=w1895, y="OPEN") -> (x .or. y?=w1896:bool)
    n1790 = case shown="True" w1896 {
      tunnel: w1895 -> [_ w2036]
      frame False {
      }
      frame True {
        n1791 = stacked-sequence {
          tunnel: w2036 -> [_ w2103 _ _]
          frame #0 {
            w2052 = "  " ("String 6")
            n1792 = local write "OPEN"(FALSE ("open")) -> ()
            n1793 = local read "string1 2"() -> (w2040:string)
            n1794 = local read "string1 3"() -> (w2039:string)
            n1795 = local read "string1 4"() -> (w2038:string)
            n1796 = property on="OPEN" class="Bool (strict)"("Visible"=FALSE) -> ()  [unwired: 2 in, 2 out]
